vi "svfa_Average Array (complex).vi"(6 "averages completed in":dbl, 7 "processing control":T1(ring), 8 "number of averages":u32=10, 9 "weighting mode":enum16{"Linear", "Exponential"}(ring), 10 "previous average array":cdb[](array[numeric]) format="%.2p", 11 "array":cdb[](array[numeric]) format="%.2p") -> (1 "averaging done":bool, 2 "averages completed out":dbl, 3 "average array":cdb[](array[numeric]) format="%.2p")   [LabVIEW 2017]
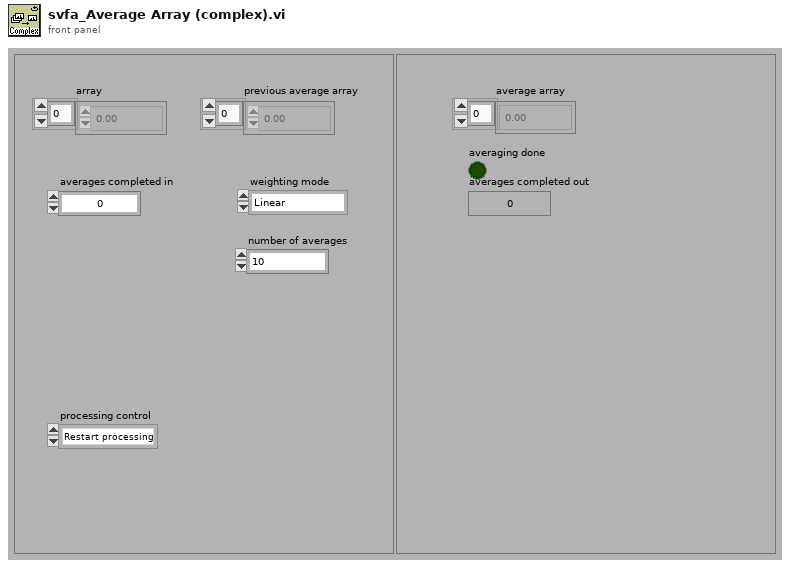
[diagram p1: front panel]
types:
  T1 = enum16{"Restart processing", "Continue processing", "Skip processing"}
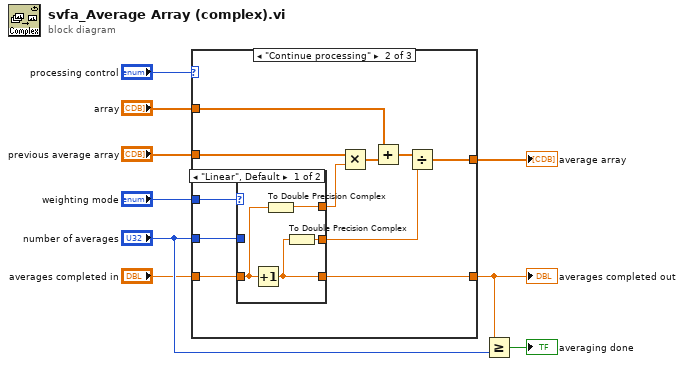
[diagram p0: block diagram]
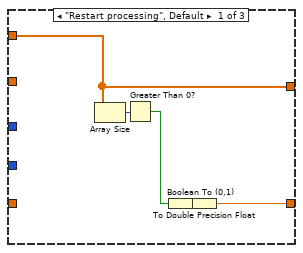
[diagram p2: hidden frame]
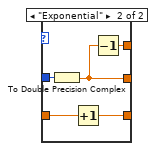
[diagram p3: hidden frame]
diagram:
  n1 = case shown="\"Continue processing\"" "processing control" {
    tunnel: "array" -> [w12 w20 _]
    tunnel: [w12 w15 w36] -> w4
    tunnel: [w10 w23 w35] -> w3
    tunnel: "previous average array" -> [_ w19 w36]
    tunnel: "number of averages" -> [_ w18 _]
    tunnel: "weighting mode" -> [_ w17 _]
    tunnel: "averages completed in" -> [_ w16 w35]
    frame "Restart processing", Default {
      n2 = Array Size(array=w12) -> (size(s)=w11:i32)
      n3 = Greater Than 0?(x=w11) -> (x > 0?=w14:bool)
      n4 = Boolean To (0,1)(Boolean=w14) -> (0, 1=w13:i16)
      n5 = To Double Precision Float(number=w13) -> (double precision float=w10:dbl)
    }
    frame "Continue processing" {
      n6 = case shown="\"Linear\", Default" w17 {
        tunnel: w16 -> [w28 w33]
        tunnel: [w26 w34] -> w23
        tunnel: [w29 w30] -> w24
        tunnel: [w27 w31] -> w22
        tunnel: w18 -> [_ w32]
        frame "Linear", Default {
          n7 = Increment(x=w28) -> (x+1=w26:dbl)
          n8 = To Double Precision Complex(1:w28) -> (0:w29:cdb)
          n9 = To Double Precision Complex(1:w26) -> (0:w27:cdb)
        }
        frame "Exponential" {
          n10 = To Double Precision Complex(1:w32) -> (0:w31:cdb)
          n11 = Increment(x=w33) -> (x+1=w34:dbl)
          n12 = Decrement(x=w31) -> (x-1=w30:cdb)
        }
      }
      n13 = Multiply(x=w19, y=w24) -> (x*y=w21:cdb[])
      n14 = Add(x=w20, y=w21) -> (x+y=w25:cdb[])
      n15 = Divide(x=w25, y=w22) -> (x/y=w15:cdb[])
    }
    frame "Skip processing" {
    }
  }
  "averages completed out" <- w3
  "average array" <- w4
  n16 = Greater Or Equal?(x=w3, y="number of averages") -> (x >= y?=→"averaging done":bool)
